vi "clear.vi"(8 "error in (no error)":errorcluster, 11 "DICT in":refnum<class "DICT.lvclass">) -> (0 "error out":errorcluster, 3 "DICT out":refnum<class "DICT.lvclass">)   [LabVIEW 2017, in "DICT.lvclass"]
uses:
  DICT.lvclass
  DICT.lvclass/DICT.ctl
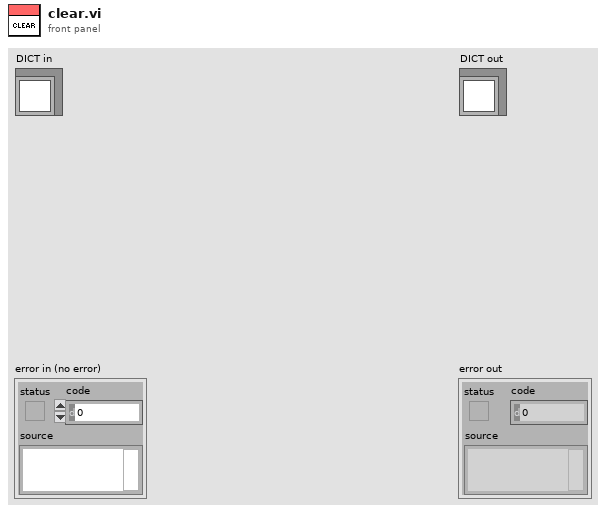
[diagram p1: front panel]
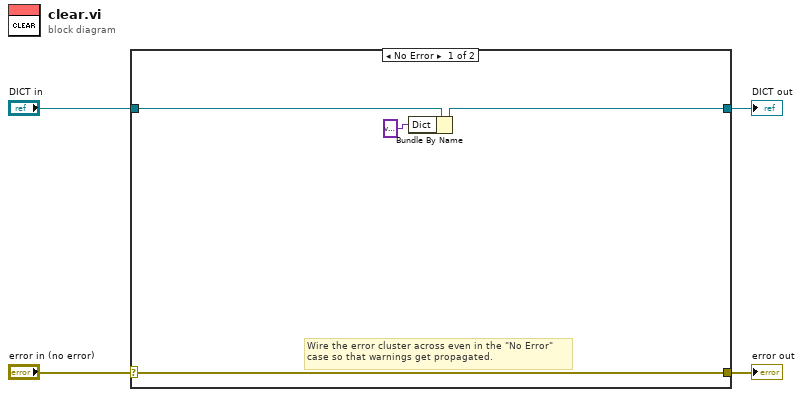
[diagram p0: block diagram]
diagram:
  n1 = case shown="No Error" "error in (no error)" {
    selector: "error in (no error)" -> [w7 w10]
    tunnel: [w7 w10] -> w3
    tunnel: [w6 w9] -> w1
    tunnel: "DICT in" -> [w8 w9]
    frame No Error {
      # "Wire the error cluster across even in the \"No Error\"\ncase so that warnings get propagated."
      n2 = Bundle By Name(cluster=w8, "Dict"=variant) -> (w6:refnum<class "DICT.lvclass">)
    }
    frame Error {
    }
  }
  "error out" <- w3
  "DICT out" <- w1
